vi "Test_sqlite3ListColumns_ListsColumns.vi"(8 "error in (no error)":errorcluster, 11 "TestCase in":refnum<class "Test sqlite3.lvclass">) -> (0 "error out":errorcluster, 3 "TestCase out":refnum<class "Test sqlite3.lvclass">)   [LabVIEW 2020, in "Test sqlite3.lvclass"]
uses:
  Test sqlite3.lvclass
  Test sqlite3.lvclass/Test sqlite3.ctl
  externals/sqlite3/Source/sqlite3.lvclass
  <vilib>/addons/_JKI Toolkits/VI Tester/TestCase.llb/TestCase.lvclass
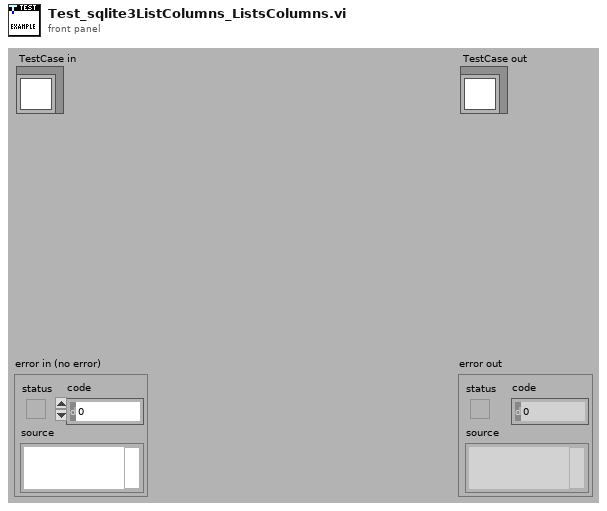
[diagram p1: front panel]
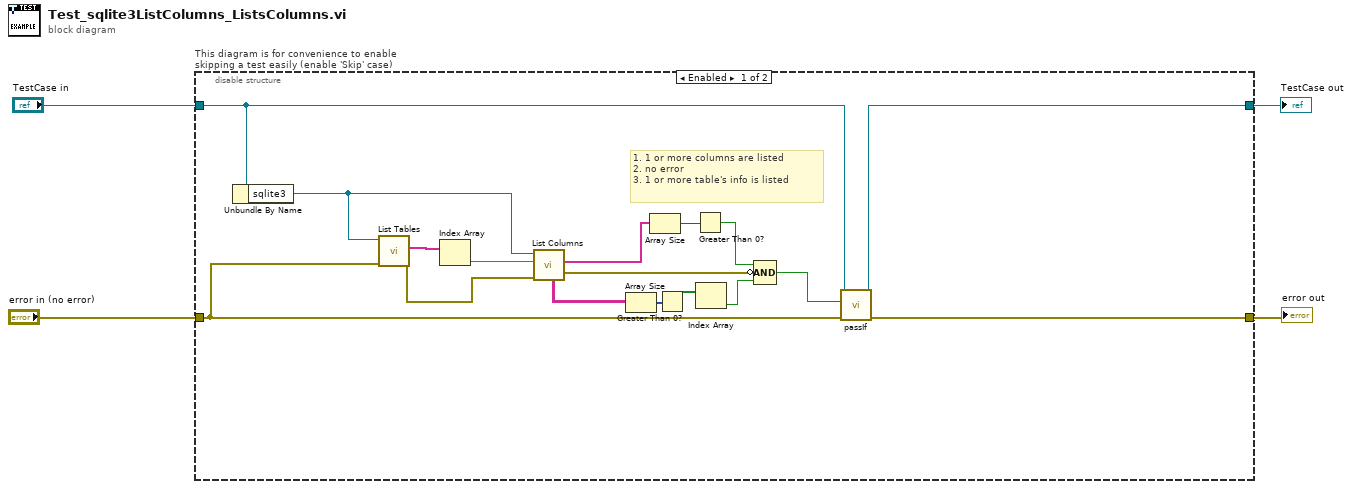
[diagram p0: block diagram]
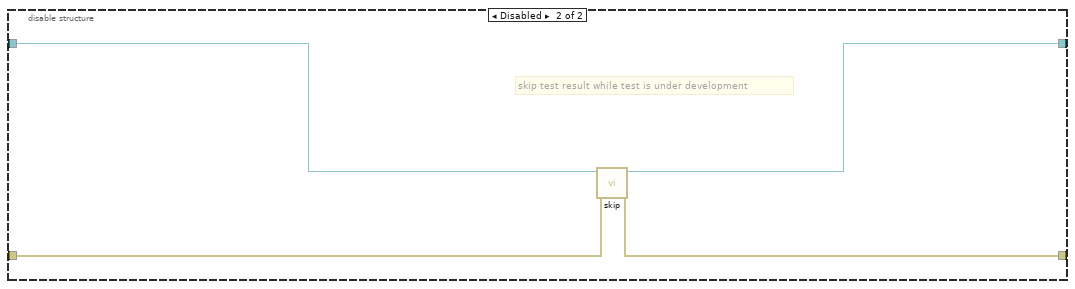
[diagram p2: hidden frame]
diagram:
  n1 = disable-structure "This diagram is for convenience to enable skipping a test easily (enable 'Skip' case)" shown="Enabled" {
    disable-tunnel: "TestCase in" -> [w19 w25]
    disable-tunnel: [w21 w23] -> w1
    disable-tunnel: [w20 w24] -> w3
    disable-tunnel: "error in (no error)" -> [w17 w22]
    frame Enabled {
      # "1. 1 or more columns are listed\n2. no error\n3. 1 or more table's info is listed"
      n2 = Unbundle By Name(w19) -> ("sqlite3"=w18:refnum<class "sqlite3.lvclass">)
      n3 = call-dynamic "List Tables.vi"("error in (no error)"=w17, "sqlite in"=w18) -> ("error out"=w16:errorcluster, "Tables out"=w15:string[])  [unwired: 7 in, 1 out]
      n4 = Index Array(array=w15) -> (element=w14:string)  [unwired: 1 in]
      n5 = call-dynamic "List Columns.vi"("error in (no error)"=w16, "Table in"=w14, "sqlite in"=w18) -> ("error out"=w8:errorcluster, "columns out"=w13:string[], "PRAGMA table info"=w10:string[][])  [unwired: 5 in, 1 out]
      n6 = Array Size(array=w10) -> (size(s)=w11:i32[])
      n7 = Array Size(array=w13) -> (size(s)=w12:i32)
      n8 = Greater Than 0?(x=w11) -> (x > 0?=w7:bool[])
      n9 = Greater Than 0?(x=w12) -> (x > 0?=w9:bool)
      n10 = Index Array(array=w7) -> (element=w6:bool)  [unwired: 1 in]
      n11 = Compound Arithmetic op=AND(w9, invert w8, w6) -> (w5:bool)
      n12 = call-dynamic "passIf.vi"("error in (no error)"=w17, "pass"=w5, "TestCase in"=w19) -> ("error out"=w20:errorcluster, "TestCase out"=w21:refnum<class "Test sqlite3.lvclass">)  [unwired: 7 in]
    }
    frame Disabled {
      # "skip test result while test is under development"
      n13 = call <vilib>:"skip.vi"("error in (no error)"=w22, "TestCase in"=w25) -> ("error out"=w24:errorcluster, "TestCase out"=w23:refnum<class "Test sqlite3.lvclass">)  [unwired: 8 in]
    }
  }
  "error out" <- w3
  "TestCase out" <- w1
